vi "svx_DAQ_SizeXControl.vi"(2 "XControl Ref":refnum<vi>, 5 "State":T2={"Channel Info Array"=[], "Timing Mode"=enum."Time", "Timing Control 1"=0.0, "Timing Control 2"=0.0, "Timing Control 3"=0, "Timing Indicator 1"=0.0, "Reference Visible?"=FALSE, "Reference Type"=enum."<none>", "Tachometer Channel"="", "Tach Pulses Per Rev"=0, "Tach Direction"=enum."CW", "Tach Slope"=enum."Rising", "Tach Threshold"=0.0, "Trigger Channel"="", "Trigger Level"=0.0, "Pretrigger Samples"=1, "Trigger Slope"=enum."Falling", "Trigger Hysteresis"=0.0, "Logging Visible?"=FALSE, "Enable Logging"=FALSE, "Logfile Path"=path "c:/test.tdms"} {"Timing Control 2" format="%#_6f"; "Channel Info Array"."Max" min=0.0 format="± %^#_4g"; "Channel Info Array"."Channel Type" items=["Voltage (V)"=0, "Charge (C)"=9, "-"=99, "SPL (Pa)"=3, "Force (lbf)"=6, "Force (N)"=1, "Acceleration (g) - IEPE"=2, "Acceleration (g) - Charge"=12, "Acceleration (g) - 4 wire DC Voltage"=22, "Velocity (in/s)"=7, "Velocity (mm/s)"=8, "Prox Probe (mil)"=4, "Prox Probe (mm)"=5]}, 9 "Reference Cluster":T1, 11 "error in (no error)":errorcluster, 12 "display state change":bool) -> (6 "State Out":T2={"Channel Info Array"=[], "Timing Mode"=enum."Time", "Timing Control 1"=0.0, "Timing Control 2"=0.0, "Timing Control 3"=0, "Timing Indicator 1"=0.0, "Reference Visible?"=FALSE, "Reference Type"=enum."<none>", "Tachometer Channel"="", "Tach Pulses Per Rev"=0, "Tach Direction"=enum."CW", "Tach Slope"=enum."Rising", "Tach Threshold"=0.0, "Trigger Channel"="", "Trigger Level"=0.0, "Pretrigger Samples"=1, "Trigger Slope"=enum."Falling", "Trigger Hysteresis"=0.0, "Logging Visible?"=FALSE, "Enable Logging"=FALSE, "Logfile Path"=path "c:/test.tdms"} caption="State" {"Timing Control 2" format="%#_6f"; "Channel Info Array"."Max" min=0.0 format="± %^#_4g"; "Channel Info Array"."Channel Type" items=["Voltage (V)"=0, "Charge (C)"=9, "-"=99, "SPL (Pa)"=3, "Force (lbf)"=6, "Force (N)"=1, "Acceleration (g) - IEPE"=2, "Acceleration (g) - Charge"=12, "Acceleration (g) - 4 wire DC Voltage"=22, "Velocity (in/s)"=7, "Velocity (mm/s)"=8, "Prox Probe (mil)"=4, "Prox Probe (mm)"=5]}, 10 "Reference Cluster Out":T1, 15 "error out":errorcluster)   [LabVIEW 2017, in "SVX NI-DAQmx AI Configuration XControl.xctl"]
uses:
  <vilib>/addons/Sound and Vibration/svt_DAQmx/Configuration XControl/SVX NI-DAQmx AI Configuration XControl.xctl
  <vilib>/addons/Sound and Vibration/svt_DAQmx/Configuration XControl/SubVIs/svx_DAQ_State.ctl
  <vilib>/addons/Sound and Vibration/svt_DAQmx/Configuration XControl/Controls/svx_DAQ_ChannelInfo.ctl
  <vilib>/addons/Sound and Vibration/svt_DAQmx/Configuration XControl/Controls/svx_DAQ_ChannelType.ctl
  <vilib>/addons/Sound and Vibration/svt_DAQmx/Configuration XControl/Controls/svx_DAQ_Coupling.ctl
  <vilib>/addons/Sound and Vibration/svt_DAQmx/Configuration XControl/Controls/svx_DAQ_Excitation.ctl
  <vilib>/addons/Sound and Vibration/svt_DAQmx/Configuration XControl/Controls/svx_DAQ_TimingType.ctl
  <vilib>/addons/Sound and Vibration/svt_DAQmx/Configuration XControl/Controls/svx_DAQ_ReferenceType.ctl
  <vilib>/addons/Sound and Vibration/svt_DAQmx/Configuration XControl/Controls/svx_DAQ_RotationDirection.ctl
  <vilib>/addons/Sound and Vibration/svt_DAQmx/Configuration XControl/Controls/svx_DAQ_Tach_Slope.ctl
  <vilib>/addons/Sound and Vibration/svt_DAQmx/Configuration XControl/Controls/svx_DAQ_Trigger_Slope.ctl
  <vilib>/addons/Sound and Vibration/svt_DAQmx/Configuration XControl/Controls/svx_DAQ_ControlRefs.ctl
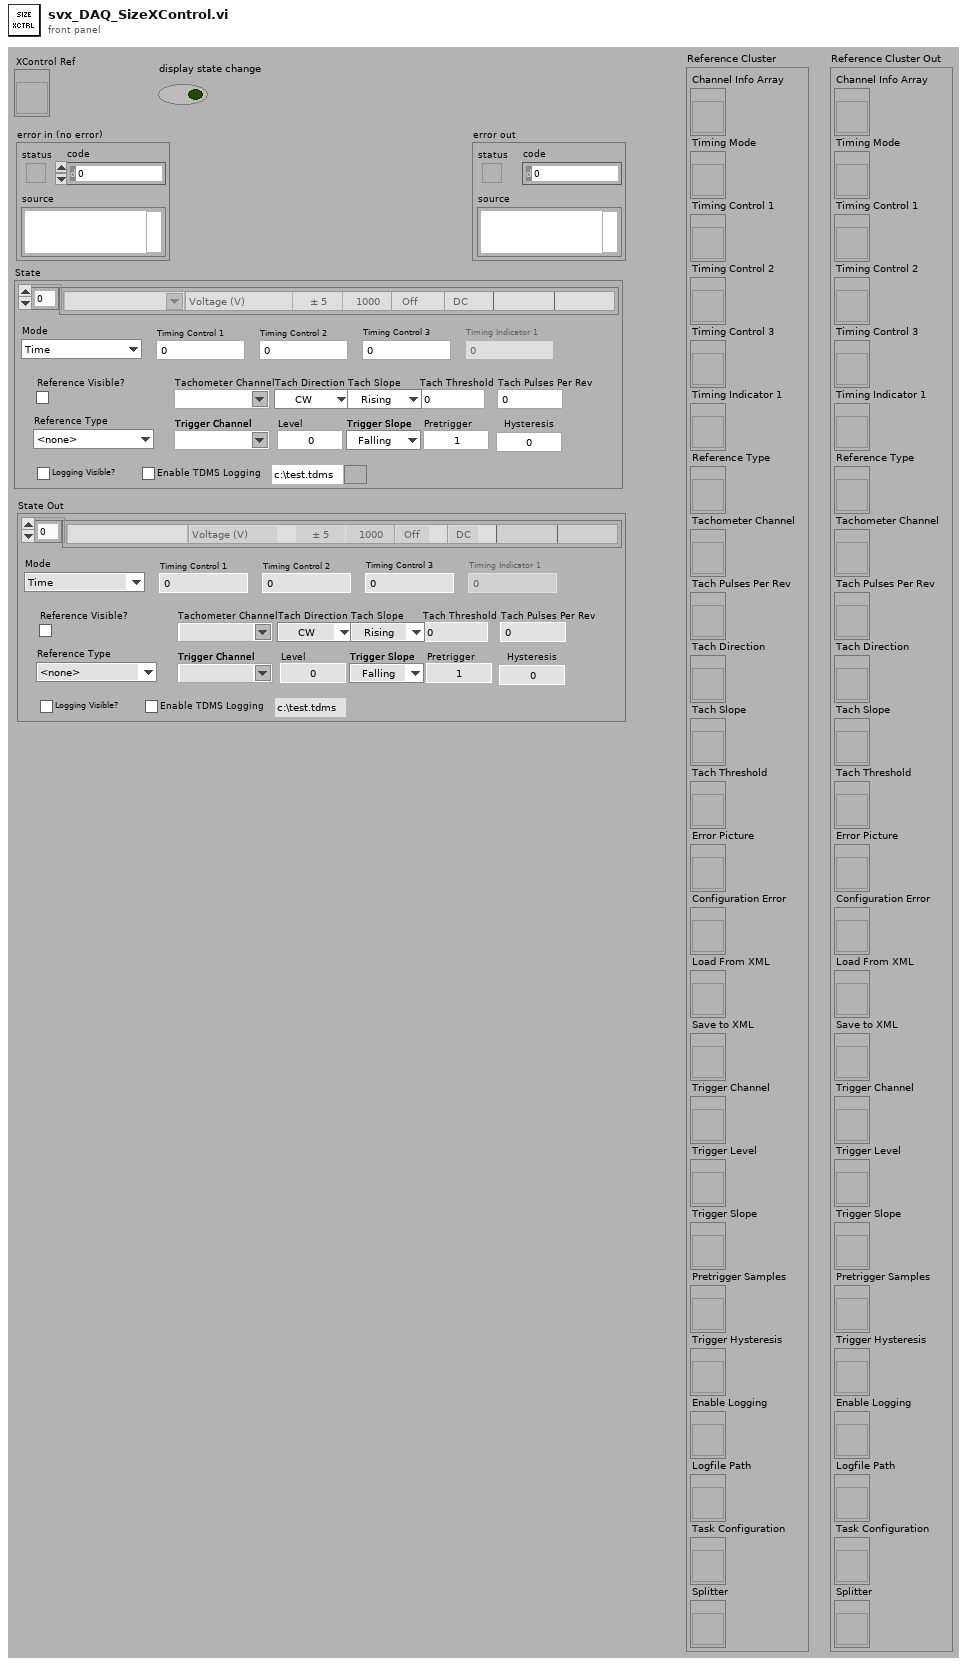
[diagram p1: front panel]
types:
  T1 = typedef "SVX NI-DAQmx AI Configuration XControl.xctl/svx_DAQ_ControlRefs.ctl" = cluster{"Channel Info Array":refnum<vi>, "Timing Mode":refnum<vi>, "Timing Control 1":refnum<vi>, "Timing Control 2":refnum<vi>, "Timing Control 3":refnum<vi>, "Timing Indicator 1":refnum<vi>, "Reference Type":refnum<vi>, "Tachometer Channel":refnum<vi>, "Tach Pulses Per Rev":refnum<vi>, "Tach Direction":refnum<vi>, "Tach Slope":refnum<vi>, "Tach Threshold":refnum<vi>, "Error Picture":refnum<vi>, "Configuration Error":refnum<vi>, "Load From XML":refnum<vi>, "Save to XML":refnum<vi>, "Trigger Channel":refnum<vi>, "Trigger Level":refnum<vi>, "Trigger Slope":refnum<vi>, "Pretrigger Samples":refnum<vi>, "Trigger Hysteresis":refnum<vi>, "Enable Logging":refnum<vi>, "Logfile Path":refnum<vi>, "Task Configuration":refnum<vi>, "Splitter":refnum<vi>}
  T2 = typedef "SVX NI-DAQmx AI Configuration XControl.xctl/svx_DAQ_State.ctl" = cluster{"Channel Info Array":T3[], "Timing Mode":T7, "Timing Control 1":dbl, "Timing Control 2":dbl, "Timing Control 3":i32, "Timing Indicator 1":dbl, "Reference Visible?":bool, "Reference Type":T8, "Tachometer Channel":string, "Tach Pulses Per Rev":i32, "Tach Direction":T9, "Tach Slope":T10, "Tach Threshold":dbl, "Trigger Channel":string, "Trigger Level":dbl, "Pretrigger Samples":i32, "Trigger Slope":T11, "Trigger Hysteresis":dbl, "Logging Visible?":bool, "Enable Logging":bool, "Logfile Path":path}
  T3 = typedef "SVX NI-DAQmx AI Configuration XControl.xctl/svx_DAQ_ChannelInfo.ctl" = cluster{"Initialized?":bool, "DAQmx Channel":tag, "Channel Type":T4, "Max":dbl, "Sensitivity":dbl, "Excitation":bool, "Coupling":T5, "Location":string, "Orientation":string, "excitation":T6}
  T4 = typedef "SVX NI-DAQmx AI Configuration XControl.xctl/svx_DAQ_ChannelType.ctl" = u16
  T5 = typedef "SVX NI-DAQmx AI Configuration XControl.xctl/svx_DAQ_Coupling.ctl" = enum16{"AC", "DC"}
  T6 = typedef "svx_DAQ_Excitation.ctl" = enum16{"Off", "Min", "Max"}
  T7 = typedef "SVX NI-DAQmx AI Configuration XControl.xctl/svx_DAQ_TimingType.ctl" = enum16{"Time", "Frequency", "Order"}
  T8 = typedef "SVX NI-DAQmx AI Configuration XControl.xctl/svx_DAQ_ReferenceType.ctl" = enum16{"<none>", "Analog Tachometer", "Analog SW Trigger"}
  T9 = typedef "SVX NI-DAQmx AI Configuration XControl.xctl/svx_DAQ_RotationDirection.ctl" = enum16{"CW", "CCW"}
  T10 = typedef "SVX NI-DAQmx AI Configuration XControl.xctl/svx_DAQ_Tach_Slope.ctl" = enum16{"Rising", "Falling"}
  T11 = typedef "SVX NI-DAQmx AI Configuration XControl.xctl/svx_DAQ_Trigger_Slope.ctl" = enum16{"Falling", "Rising"}
  T12 = enum16{"Sticks Top/Left", "Sticks Bottom/Right", "Proportional"}
  T13 = typedef "LVPointTypeDef.ctl" = cluster{"Horizontal":i16, "Vertical":i16}
  T14 = typedef "LVBoundsTypeDef.ctl" = cluster{"Width":u32, "Height":u32}
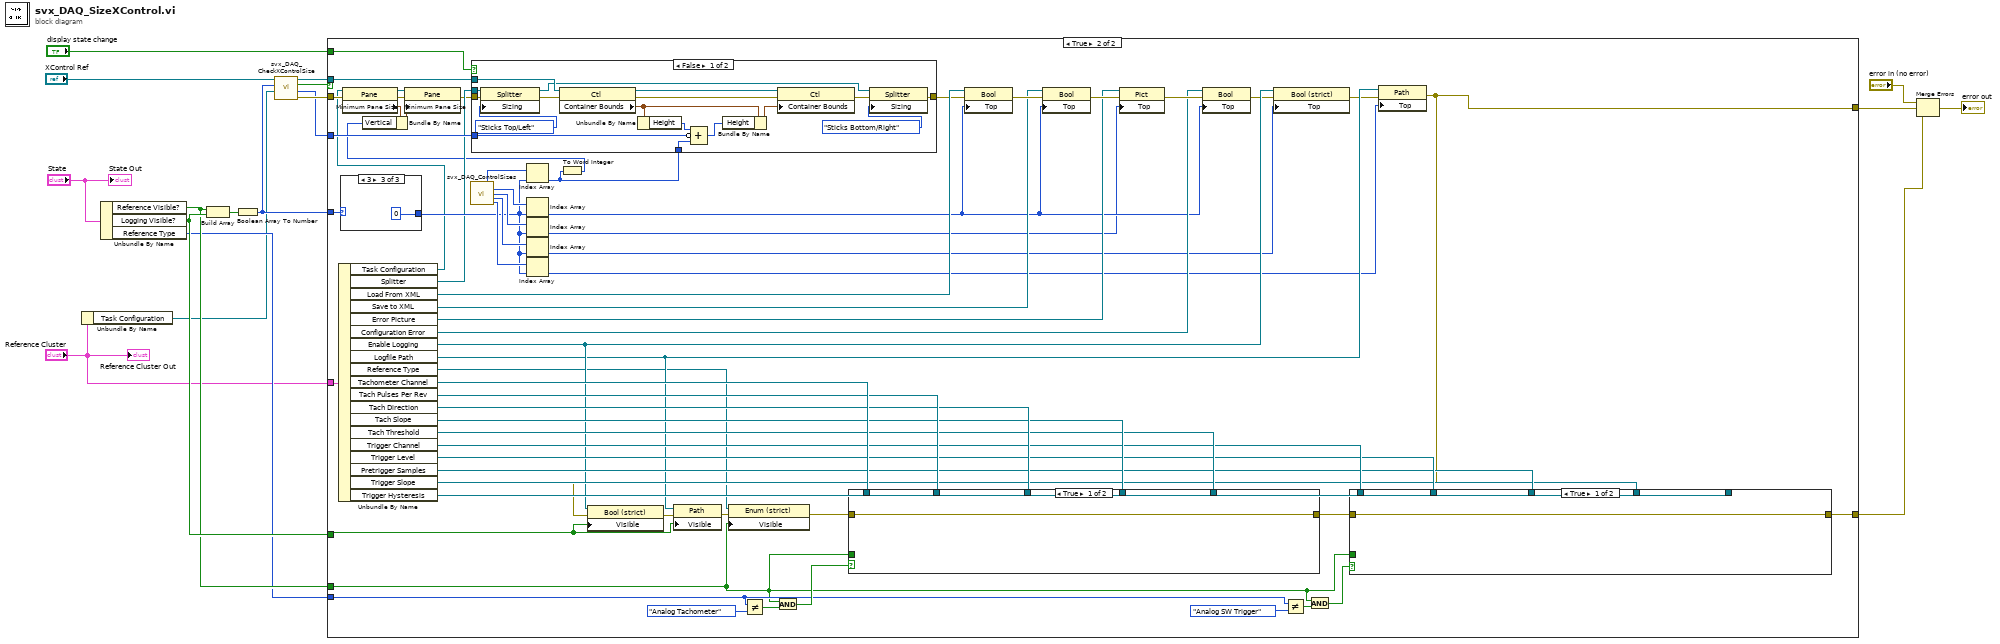
[diagram p0: block diagram]
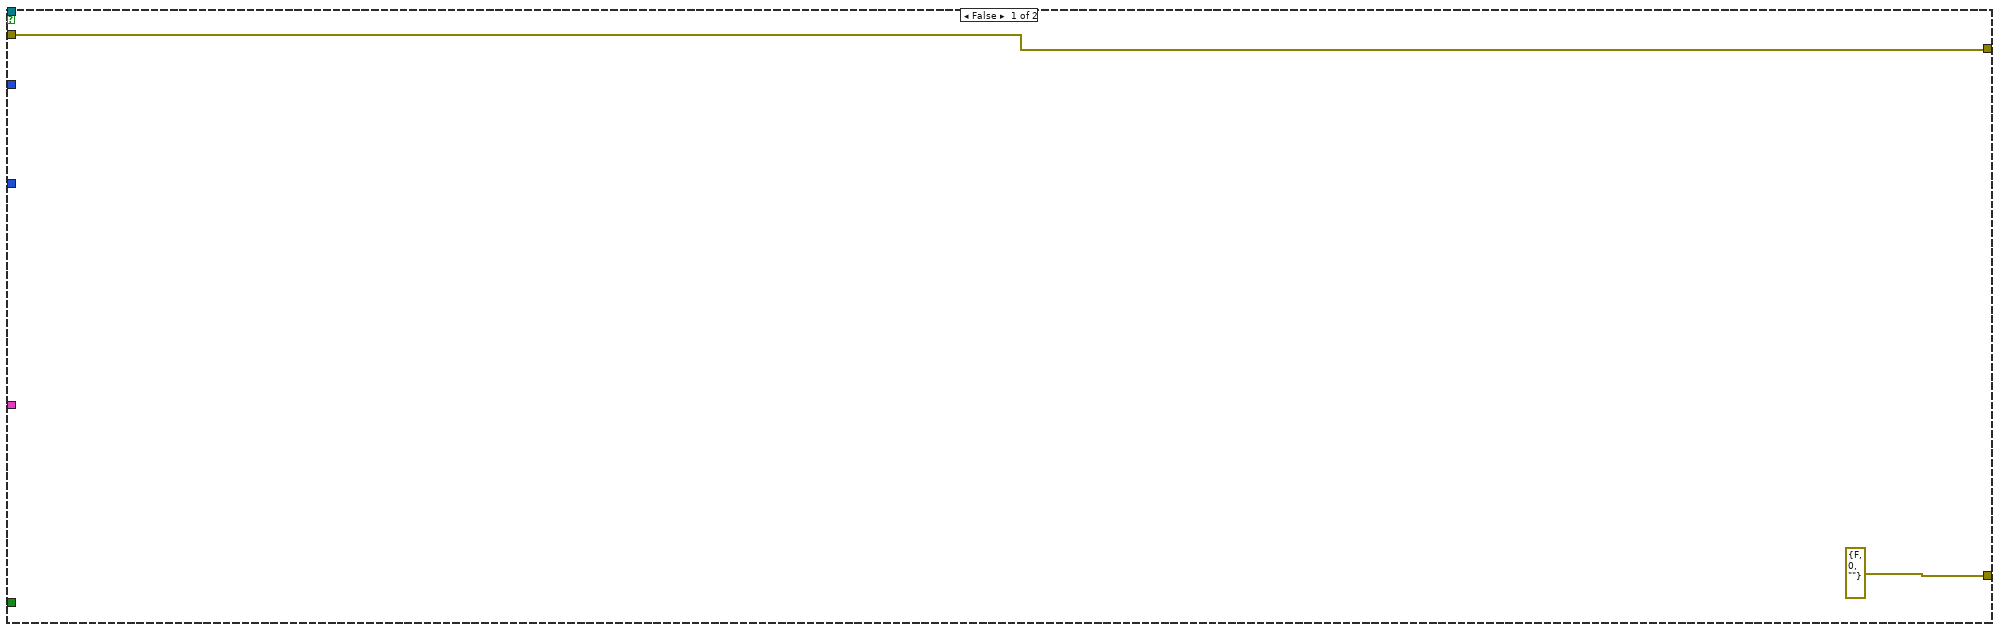
[diagram p2: hidden frame]
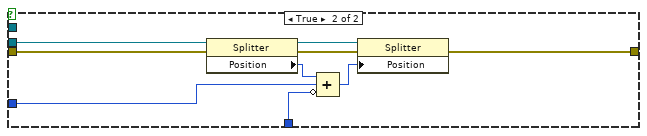
[diagram p3: hidden frame]
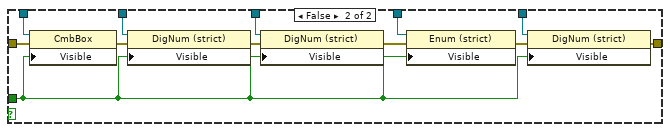
[diagram p4: hidden frame]
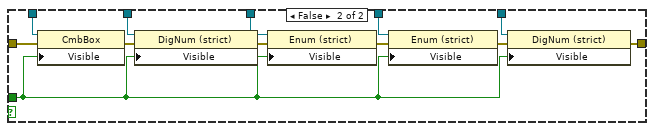
[diagram p5: hidden frame]
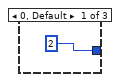
[diagram p6: hidden frame]
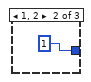
[diagram p7: hidden frame]
diagram:
  n1 = Unbundle By Name("Reference Cluster") -> ("Task Configuration"=w3:refnum<vi>)
  n2 = Unbundle By Name("State") -> ("Reference Visible?"=w7:bool, "Logging Visible?"=w8:bool, "Reference Type"=w5:T8)
  n3 = Build Array(w7, w8) -> (w11:bool[])
  n4 = Boolean Array To Number(Boolean array=w11) -> (number=w9:u32)
  n5 = call <vilib>:"svx_DAQ_CheckXControlSize.vi"("Task Configuration Pane"=w3, "XControl Boolean Size Number"=w9, "XControl Ref"="XControl Ref") -> ("error out"=w16:errorcluster, "Task Configuration Pane Height"=w2:u32, "Update Size?"=w12:bool, "XControl Ref Out"=w17:refnum<vi>)  [unwired: 3 in]
  n6 = case shown="True" w12 {
    tunnel: w17 -> [_ w36]
    tunnel: w16 -> [w20 w24]
    tunnel: [w20 w48] -> w14
    tunnel: "Reference Cluster" -> [_ w83]
    tunnel: w9 -> [_ w75]
    tunnel: w8 -> [_ w74]
    tunnel: w7 -> [_ w37]
    tunnel: [errorcluster {"status"=FALSE, "code"=0, "source"=""} ("error out") w62] -> w6
    tunnel: w5 -> [_ w41]
    tunnel: w2 -> [_ w33]
    tunnel: "display state change" -> [_ w32]
    frame False {
    }
    frame True {
      n7 = Unbundle By Name(w83) -> ("Task Configuration"=w21:refnum<vi>, "Splitter"=w31:refnum<vi>, "Load From XML"=w79:refnum<vi>, "Save to XML"=w78:refnum<vi>, "Error Picture"=w77:refnum<vi>, "Configuration Error"=w76:refnum<vi>, "Enable Logging"=w57:refnum<vi>, "Logfile Path"=w56:refnum<vi>, "Reference Type"=w47:refnum<vi>, "Tachometer Channel"=w73:refnum<vi>, "Tach Pulses Per Rev"=w72:refnum<vi>, "Tach Direction"=w71:refnum<vi>, "Tach Slope"=w70:refnum<vi>, "Tach Threshold"=w69:refnum<vi>, "Trigger Channel"=w68:refnum<vi>, "Trigger Level"=w67:refnum<vi>, "Pretrigger Samples"=w66:refnum<vi>, "Trigger Slope"=w65:refnum<vi>, "Trigger Hysteresis"=w64:refnum<vi>)
      n8 = case shown="3" w75 {
        tunnel: [2 ("index") 1 ("index") 0 ("index")] -> w34
        frame 0, Default {
        }
        frame 1, 2 {
        }
        frame 3 {
        }
      }
      n9 = property class="Pane"(reference=w21, error in=w24) -> (reference out=w30:refnum<vi>, error out=w29:errorcluster, "Minimum Pane Size"=w28:T13)
      n10 = call <vilib>:"svx_DAQ_ControlSizes.vi"() -> ("Task Configuration Pane Heights"=w35:u32[], "Buttons Top - Pixel Values"=w61:i32[], "Error Image Top - Pixel Values"=w60:i32[], "Enable Logging Top - Pixel Values"=w53:i32[], "Logfile Path Top - Pixel Values"=w52:i32[])  [unwired: 10 in, 1 out]
      n11 = Index Array(array=w35, index=w34) -> (element=w22:u32)
      n12 = Index Array(array=w61, index=w34) -> (element=w59:i32)
      n13 = Index Array(array=w60, index=w34) -> (element=w58:i32)
      n14 = Index Array(array=w53, index=w34) -> (element=w51:i32)
      n15 = Index Array(array=w52, index=w34) -> (element=w50:i32)
      n16 = To Word Integer(number=w22) -> (16bit integer=w26:i16)
      n17 = Bundle By Name(cluster=w28, "Vertical"=w26) -> (w27:T13)
      n18 = property class="Pane"(reference=w30, error in=w29, "Minimum Pane Size"=w27) -> (error out=w23:errorcluster)  [unwired: 1 out]
      n19 = case shown="False" w32 {
        tunnel: w36 -> [w100 _]
        tunnel: w33 -> [w94 w103]
        tunnel: w22 -> [w93 w102]
        tunnel: w31 -> [w91 w108]
        tunnel: w23 -> [w90 w107]
        tunnel: [w87 w109] -> w25
        frame False {
          n20 = property class="Splitter"(reference=w91, error in=w90, "Sizing"=T12."Sticks Top/Left") -> (reference out=w88:refnum<vi>, error out=w89:errorcluster)
          n21 = property class="Ctl"(reference=w100, error in=w89) -> (reference out=w99:refnum<vi>, error out=w98:errorcluster, "Container Bounds"=w96:T14)
          n22 = Unbundle By Name(w96) -> ("Height"=w95:u32)
          n23 = Compound Arithmetic op=ADD(w95, invert w94, w93) -> (w92:u32)
          n24 = Bundle By Name(cluster=w96, "Height"=w92) -> (w97:T14)
          n25 = property class="Ctl"(reference=w99, error in=w98, "Container Bounds"=w97) -> (error out=w86:errorcluster)  [unwired: 1 out]
          n26 = property class="Splitter"(reference=w88, error in=w86, "Sizing"=T12."Sticks Bottom/Right") -> (error out=w87:errorcluster)  [unwired: 1 out]
        }
        frame True {
          n27 = property class="Splitter"(reference=w108, error in=w107) -> (reference out=w106:refnum<vi>, error out=w105:errorcluster, "Position"=w104:i32)
          n28 = Compound Arithmetic op=ADD(w104, w103, invert w102) -> (w101:u32)
          n29 = property class="Splitter"(reference=w106, error in=w105, "Position"=w101) -> (error out=w109:errorcluster)  [unwired: 1 out]
        }
      }
      n30 = Not Equal?(x=w41, y=svx_DAQ_ReferenceType."Analog Tachometer") -> (x != y?=w38:bool)
      n31 = And(x=w37, y=w38) -> (x .and. y?=w44:bool)
      n32 = property class="Bool"(reference=w79, error in=w25, "Top"=w59) -> (error out=w81:errorcluster)  [unwired: 1 out]
      n33 = property class="Bool"(reference=w78, error in=w81, "Top"=w59) -> (error out=w80:errorcluster)  [unwired: 1 out]
      n34 = property class="Pict"(reference=w77, error in=w80, "Top"=w58) -> (error out=w82:errorcluster)  [unwired: 1 out]
      n35 = property class="Bool"(reference=w76, error in=w82, "Top"=w59) -> (error out=w55:errorcluster)  [unwired: 1 out]
      n36 = property class="Bool (strict)"(reference=w57, error in=w55, "Top"=w51) -> (error out=w54:errorcluster)  [unwired: 1 out]
      n37 = Not Equal?(x=w41, y=svx_DAQ_ReferenceType."Analog SW Trigger") -> (x != y?=w40:bool)
      n38 = And(x=w37, y=w40) -> (x .and. y?=w39:bool)
      n39 = property class="Path"(reference=w56, error in=w54, "Top"=w50) -> (error out=w48:errorcluster)  [unwired: 1 out]
      n40 = property class="Bool (strict)"(reference=w57, error in=w48, "Visible"=w74) -> (error out=w49:errorcluster)  [unwired: 1 out]
      n41 = property class="Path"(reference=w56, error in=w49, "Visible"=w74) -> (error out=w46:errorcluster)  [unwired: 1 out]
      n42 = property class="Enum (strict)"(reference=w47, error in=w46, "Visible"=w37) -> (error out=w45:errorcluster)  [unwired: 1 out]
      n43 = case shown="True" w44 {
        tunnel: w73 -> [_ w135]
        tunnel: w72 -> [_ w134]
        tunnel: w71 -> [_ w133]
        tunnel: w70 -> [_ w132]
        tunnel: w69 -> [_ w131]
        tunnel: [w123 w126] -> w63
        tunnel: w37 -> [_ w125]
        tunnel: w45 -> [w123 w124]
        frame True {
        }
        frame False {
          n44 = property class="CmbBox"(reference=w135, error in=w124, "Visible"=w125) -> (error out=w130:errorcluster)  [unwired: 1 out]
          n45 = property class="DigNum (strict)"(reference=w134, error in=w130, "Visible"=w125) -> (error out=w129:errorcluster)  [unwired: 1 out]
          n46 = property class="Enum (strict)"(reference=w133, error in=w129, "Visible"=w125) -> (error out=w128:errorcluster)  [unwired: 1 out]
          n47 = property class="Enum (strict)"(reference=w132, error in=w128, "Visible"=w125) -> (error out=w127:errorcluster)  [unwired: 1 out]
          n48 = property class="DigNum (strict)"(reference=w131, error in=w127, "Visible"=w125) -> (error out=w126:errorcluster)  [unwired: 1 out]
        }
      }
      n49 = case shown="True" w39 {
        tunnel: w68 -> [_ w122]
        tunnel: w67 -> [_ w121]
        tunnel: w66 -> [_ w120]
        tunnel: w65 -> [_ w119]
        tunnel: w64 -> [_ w118]
        tunnel: w63 -> [w110 w117]
        tunnel: [w110 w112] -> w62
        tunnel: w37 -> [_ w111]
        frame True {
        }
        frame False {
          n50 = property class="CmbBox"(reference=w122, error in=w117, "Visible"=w111) -> (error out=w116:errorcluster)  [unwired: 1 out]
          n51 = property class="DigNum (strict)"(reference=w121, error in=w116, "Visible"=w111) -> (error out=w115:errorcluster)  [unwired: 1 out]
          n52 = property class="DigNum (strict)"(reference=w120, error in=w115, "Visible"=w111) -> (error out=w114:errorcluster)  [unwired: 1 out]
          n53 = property class="Enum (strict)"(reference=w119, error in=w114, "Visible"=w111) -> (error out=w113:errorcluster)  [unwired: 1 out]
          n54 = property class="DigNum (strict)"(reference=w118, error in=w113, "Visible"=w111) -> (error out=w112:errorcluster)  [unwired: 1 out]
        }
      }
    }
  }
  n55 = Merge Errors("error in (no error)", w14, w6) -> (→"error out":errorcluster)
  "State Out" <- "State"
  "Reference Cluster Out" <- "Reference Cluster"
